vi "Calculate Scale.vi"(10 "FoV":dbl, 11 "Image Resolution":i32) -> (3 "Scale":dbl)   [LabVIEW 2012]
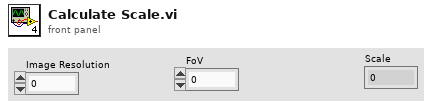
[diagram p1: front panel]
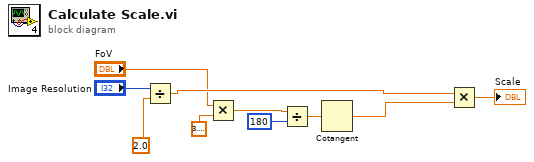
[diagram p0: block diagram]
diagram:
  n1 = Divide(x="Image Resolution", y=2.0) -> (x/y=w8:dbl)
  n2 = Multiply(x="FoV", y=3.141592653589793) -> (x*y=w5:dbl)
  n3 = Divide(x=w5, y=180) -> (x/y=w4:dbl)
  n4 = Cotangent(1:w4) -> (0:w2:dbl)
  n5 = Multiply(x=w8, y=w2) -> (x*y=→"Scale":dbl)
